vi "graph_builder.vi"(2 "Voltage StdDev Graph in":T1(array[cluster]), 3 "Voltage 1":dbl, 4 "Voltage Graph in":cluster{"x values":dbl[], "voltages":dbl[]}[](array[cluster]), 5 "Voltage StdDev 2":dbl, 6 "Voltage StdDev 1":dbl, 7 "Voltage 2":dbl) -> (0 "Voltage StdDev Graph out":T1(array[cluster]), 1 "Voltage Graph out":cluster{"x values":dbl[], "voltages":dbl[]}[](array[cluster]))   [LabVIEW 2010]
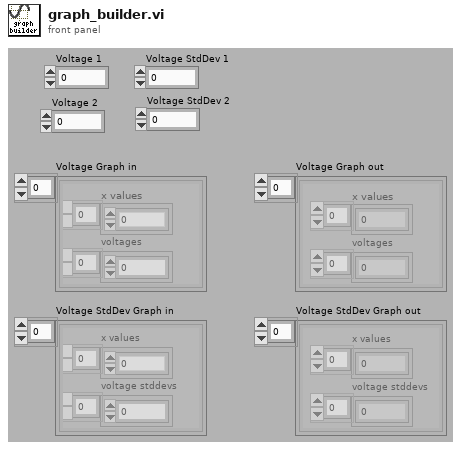
[diagram p1: front panel]
types:
  T1 = cluster{"x values":dbl[], "voltage stddevs":dbl[]}[]
  T2 = cluster{"x values":dbl[], "voltage stddevs":dbl[]}
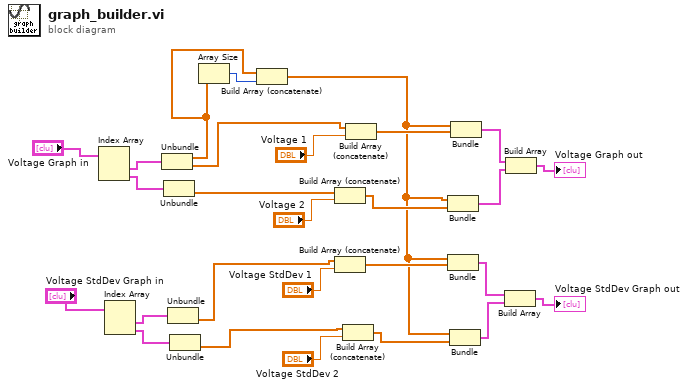
[diagram p0: block diagram]
diagram:
  n1 = Index Array(array="Voltage Graph in") -> (element #1=w18:cluster{"x values":dbl[], "voltages":dbl[]}, element #2=w17:cluster{"x values":dbl[], "voltages":dbl[]})  [unwired: 2 in]
  n2 = Index Array(array="Voltage StdDev Graph in") -> (element #1=w11:T2, element #2=w10:T2)  [unwired: 2 in]
  n3 = Unbundle(w18) -> ("x values"=w15:dbl[], "voltages"=w13:dbl[])
  n4 = Unbundle(w17) -> ("voltages"=w12:dbl[])  [unwired: 1 out]
  n5 = Unbundle(w11) -> ("voltage stddevs"=w8:dbl[])  [unwired: 1 out]
  n6 = Unbundle(w10) -> ("voltage stddevs"=w7:dbl[])  [unwired: 1 out]
  n7 = Array Size(array=w15) -> (size(s)=w16:i32)
  n8 = Build Array (concatenate)(w15, w16) -> (w14:dbl[])
  n9 = Build Array (concatenate)(w12, "Voltage 2") -> (w22:dbl[])
  n10 = Build Array (concatenate)(w8, "Voltage StdDev 1") -> (w21:dbl[])
  n11 = Build Array (concatenate)(w7, "Voltage StdDev 2") -> (w20:dbl[])
  n12 = Build Array (concatenate)(w13, "Voltage 1") -> (w23:dbl[])
  n13 = Bundle(w14, w22) -> (w5:cluster{dbl[], dbl[]})  [unwired: 1 in]
  n14 = Bundle(w14, w21) -> (w4:cluster{dbl[], dbl[]})  [unwired: 1 in]
  n15 = Bundle(w14, w20) -> (w3:cluster{dbl[], dbl[]})  [unwired: 1 in]
  n16 = Bundle(w14, w23) -> (w6:cluster{dbl[], dbl[]})  [unwired: 1 in]
  n17 = Build Array(w4, w3) -> (→"Voltage StdDev Graph out":cluster{dbl[], dbl[]}[])
  n18 = Build Array(w6, w5) -> (→"Voltage Graph out":cluster{dbl[], dbl[]}[])
